vi "PH_SHS_Analysis_Calibrator.contents.vi"   [LabVIEW 2014, in "PH_SHS_Analysis_Calibrator.lvlib"]
doc: "This class takes and stores several beam profile settings. This is relevant for the class PH_ImageOperator.\n\nThis class is part of the PHELIX user layer."
uses:
  PH_SHS_Analysis_Calibrator.lvlib
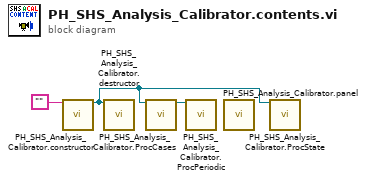
[diagram p0: block diagram]
diagram:
  n1 = call "PH_SHS_Analysis_Calibrator.constructor.vi"("name"="") -> ("i ref out"=w1:refnum<vi>)  [unwired: 16 in, 2 out]
  n2 = call "PH_SHS_Analysis_Calibrator.destructor.vi"("i ref in"=w1) -> ()  [unwired: 18 in, 1 out]
  n3 = call "PH_SHS_Analysis_Calibrator.ProcCases.vi"("i ref in"=w1) -> ("i ref out"=w3:refnum<vi>)  [unwired: 16 in, 2 out]
  n4 = call "PH_SHS_Analysis_Calibrator.ProcPeriodic.vi"("i ref in"=w3) -> ()  [unwired: 16 in, 3 out]
  n5 = call "PH_SHS_Analysis_Calibrator.panel.vi"() -> ()  [unwired: 19 in, 1 out]
  n6 = call "PH_SHS_Analysis_Calibrator.ProcState.vi"("i ref in"=w1) -> ()  [unwired: 16 in, 3 out]
